vi "ExtractLoopsFromDrawI32WithSaveTST SAve2.vi"() -> ()   [LabVIEW 2018]
uses:
  <vilib>/vision/Image Controls.llb/IMAQ Image.ctl
  GlobalArrayLoops.vi
  <vilib>/vision/NI_Vision_Development_Module.lvlib
  <vilib>/ptbypt/NI_PtbyPt.lvlib
  <vilib>/Analysis/NI_AALBase.lvlib
panel:
  in  "Delay":dbl
  in  "AppendName":string
  in  "Constant":dbl=2.0 format="%.2f"
  in  "# Shifts":i32 min=0 max=8 step=1
  out "Image Out":T1
  in  "Initialize":bool
  in  "Image shift Y":i16
  in  "Image shift X":i16
  in  "Rot of image (deg)":sgl format="%.2f"
  in  "Normalize?":bool
  in  "Export All loops":bool
  in  "Shift Brightness?":bool
  in  "Enhance contrast?":bool
  in  "process loops?":bool=TRUE
  in  "Data Shift (bits)":i32=32768
  in  "Optional Rectangle":i32[](array[numeric])
  in  "Offset":dbl
  in  "SubtractBackground":bool
  in  "SaveBackground":bool
  in  "Save Button":bool
  out "CentersY":dbl[](array[numeric])
  out "CentersX":dbl[](array[numeric])
  in  "expAll":bool
  in  "exp":bool
  in  "contrast":dbl=1.0 format="%.2f"
  in  "Shift bright":dbl format="%.2f"
  out "ROI":T2
  out "Other Parameters":sgl[](array[numeric])
  out "Coordinates":i32[](array[numeric])
  in  "Loop stretch factor":dbl=15.0
  in  "Overlay loops!":bool
  out "Waveform Graph":dbl[][](graph)
  out "Coercive field  array":dbl[](array[numeric])
  out "Saturation array":dbl[](array[numeric])
  out "element":path
  out "BField":dbl[](array[numeric])
  in  "quadratic":dbl
  in  "Artificial x axis":bool
  in  "Faraday":dbl
  out "Remanence array":dbl[](array[numeric])=[-0.6665042042732239, -0.6516115069389343, -0.6760320067405701, -0.7227444648742676, 0.9848632216453552, 0.9883291125297546, 0.9750781655311584, 0.9934242963790894, 0.998292863368988, 0.9937769174575806, 0.9914392828941345, 0.9886137247085571, 0.9929239749908447, 0.9905381798744202, 0.988884687423706, 0.9859522581100464]
  out "ArrayLoops":dbl[][](array[numeric])=[[-8.399140210504821e+16, -6.383327329538546e+16, -7.300137106498384e+16, -7.299504888063269e+16, -7.545170145583659e+16, -6.992078814201549e+16, -8.44639172329355e+16, -1.3869430462570203e+17, -1.940946935865587e+17, -2.6899589959241552e+17, -3.841794265110722e+18, -3.5900544809762724e+18, -3.6362559596608225e+18, -3.50006165326631e+18, -3.327418536555498e+18, -3.784010531202494e+18, -3.449798578704159e+18, -3.328924867465459e+18, -3.311856048910509e+18, -3.4747904779405885e+18, -3.363990492336348e+18, -3.5235450226296233e+18, -3.5302608397729183e+18, -3.312218887780462e+18, -3.018598705633053e+18, -2.597754032832259e+18, -1.6360642472216494e+18, -1.0784516950489162e+17, -9.602954260961573e+16, -6.323074092330715e+16, -7.149779705137957e+16, -6.551521684505044e+16, -7.017147678836868e+16, -5.66990233766953e+16, -7.36723480449653e+16, 9.06092203023e-312, 2.141114181e-314, 2.4380364662986284e-231, 9.346337195181631e+20, 1.633936759043e-312, 8.184566024846808e-246, 3.441969216927865e-231, 1.8079404139024e-311, 5.8225571452e-313, 7.0610898928135075e-248, 5.749237705750308e-237, 2.80802498703826e-272, 4.45619116103e-313, 1.9118376e-316, 1.08168262e-315, 1.2469008049271105e+190, 5.335e-320, 3.18299368694e-313, 5.3527994774636694e+112, 1.4981290295104e-311, 1.6e-322, 2.1219957984e-314, 1.1251988247307957e-242, 3.1959050680695386e-231, 6.491120506e-315, 7.6391848542e-313, 2.3e-322, 1.455191297151144e-297, 2.1734535962868656e-66, 4.15911175029e-312, 5.995413155e-315, 3.18299368645e-313, 0.0, 1.1251988247307907e-242, 1.706694794319977e-138]]
  in  "n":i32=17
  out "XY Graph":cluster{"BField":dbl[], dbl[]}(graph)
  in  "Index of structure":i32
  in  "Array curves":dbl[][](array[numeric])=[[1.2468077718936927e+32, 1.1436107690770144e+32, 1.622459903179132e+32, 1.5181185795245691e+32, 2.0453528136560583e+32, 2.0512036276842735e+32, 2.9457901653443808e+32, 2.6269200225087976e+32, 1.193618727e-315, 2.1814116731123e-311, 1.032625499241048e-305, 7.46947828771e-312, 7.46942518498e-312, 8.1e-322, 8.289046e-317, 0.0]]
  out "Array":sgl[](array[numeric])=[20196.236, 20196.082, 20275.379, 20237.95, 19425.816, 19220.783, 19457.14, 19034.357, 18600.703, 18844.629, 18578.557, 18244.92, 17575.152, 17728.125, 17648.24, 17715.977]
  in  "Go through all images at one rot.":bool
  in  "stop":bool
  out "Image":T1(plugin-control)
  in  "index":i32(slide)=70 min=-1 max=160 step=1 scale=0.0..160.0
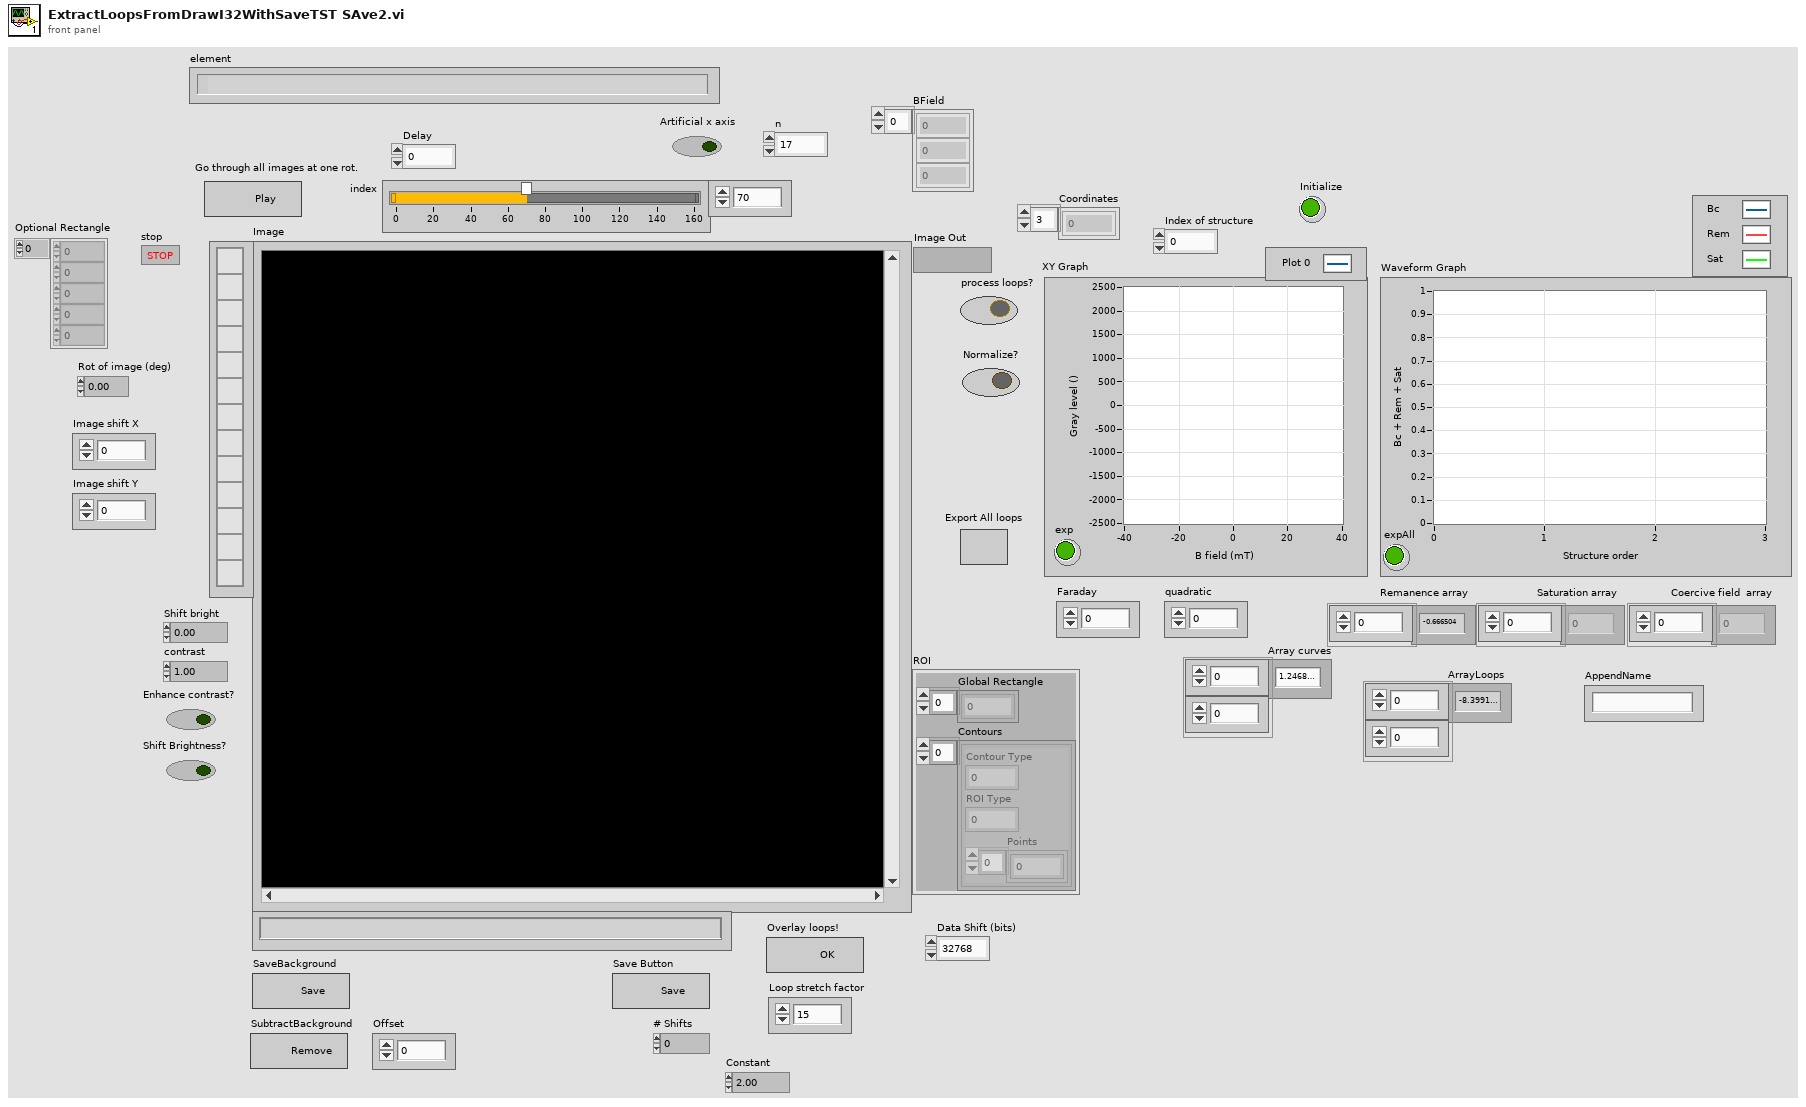
[diagram p1: front panel]
types:
  T1 = typedef "IMAQ Image.ctl" = refnum<image>
  T2 = cluster{"Global Rectangle":i32[], "Contours":cluster{"Contour Type":u32, "ROI Type":u32, "Points":i32[]}[]}
  T3 = typedef "Image Type" = u32
  T4 = cluster{"Desired Font (Application)":enum16{"User-specified Font", "Application Font", "System Font", "Dialog Font"}, "[User-specified Font]":cluster{"Font Name":string, "Size":i16, "Strikeout?":bool, "Italic?":bool, "Underline?":bool, "Outline?":bool, "Shadow?":bool, "Bold?":bool, "Rotation Angle":dbl}, "Horizontal Alignment":i16, "Vertical Alignment":i16}
  T5 = cluster{"Contour Type":u32, "ROI Type":u32, "Points":i32[]}[]
  T6 = cluster{"Global Rectangle":i32[], cluster{"Contour Type":u32, "ROI Type":u32, "Points":i32[]}[]}
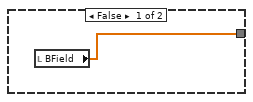
[diagram p6: hidden frame]
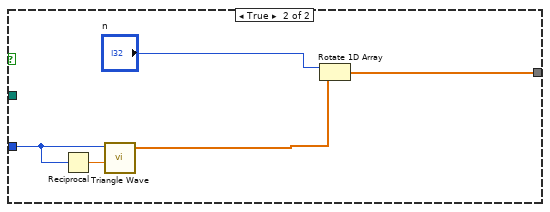
[diagram p7: hidden frame]
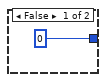
[diagram p9: hidden frame]
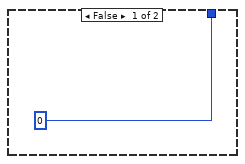
[diagram p13: hidden frame]
diagram:
  w5 = T3 1 items=["Grayscale (U8)", "Grayscale (I16)", "Grayscale (SGL)", "Complex (CSG)", "RGB (U32)", "HSL (U32)", "RGB (U64)", "Grayscale (U16)"] ("Image Type")
  w8 = T3 1 items=["Grayscale (U8)", "Grayscale (I16)", "Grayscale (SGL)", "Complex (CSG)", "RGB (U32)", "HSL (U32)", "RGB (U64)", "Grayscale (U16)"] ("Image Type")
  w12 = T3 1 items=["Grayscale (U8)", "Grayscale (I16)", "Grayscale (SGL)", "Complex (CSG)", "RGB (U32)", "HSL (U32)", "RGB (U64)", "Grayscale (U16)"] ("Image Type")
  w23 = T3 0 items=["Grayscale (U8)", "Grayscale (I16)", "Grayscale (SGL)", "Complex (CSG)", "RGB (U32)", "HSL (U32)", "RGB (U64)", "Grayscale (U16)"] ("Image Type")
  w26 = T3 7 items=["Grayscale (U8)", "Grayscale (I16)", "Grayscale (SGL)", "Complex (CSG)", "RGB (U32)", "HSL (U32)", "RGB (U64)", "Grayscale (U16)"] ("Image Type")
  n1 = call "File Dialog2"() -> ("selected path"=w18:path)  [unwired: 12 in, 3 out]
  n2 = disable-structure shown="Disabled" {
    disable-tunnel: [w33 _] -> _
    frame Disabled {
      n3 = call "File Dialog"() -> ("selected paths"=w33:path[])  [unwired: 12 in, 3 out]
    }
    frame Enabled {
    }
  }
  n4 = List Folder(path=w18, pattern="*.png") -> (path out=w17:path, filenames=w16:string[])  [unwired: 2 in, 2 out]
  n5 = for {
    tunnel: [w37] -> w15 mode=indexing if=w34
    tunnel: w17 -> [w38]
    tunnel: w16 -> [w36] mode=indexing
    n6 = Not Equal?(x=w36, y="mask.png") -> (x != y?=w34:bool)
    n7 = Build Path(base path=w38, name or relative path=w36) -> (appended path=w37:path)
  }
  n8 = Array Size(array=w15) -> (size(s)=w3:i32)
  n9 = List Folder(path=w18, pattern="*.txt") -> (path out=w13:path, filenames=w21:string[])  [unwired: 2 in, 2 out]
  n10 = Decrement(x=w3) -> (x-1=w1:i32)
  n11 = call "IMAQ Create"("Image Name"="sub", "Image Type"=w8) -> ("New Image"=w7:T1)  [unwired: 3 in, 1 out]
  n12 = property on="index" class="Slide (strict)"("Maximum"=w1) -> ()  [unwired: 2 in, 2 out]
  n13 = Index Array(array=w21) -> (element=w20:string)  [unwired: 1 in]
  n14 = property on="index" class="Slide (strict)"("Scale.Maximum"=w1) -> ()  [unwired: 2 in, 2 out]
  n15 = call "IMAQ Create"("Image Name"="Baxck", "Image Type"=w12) -> ("New Image"=w10:T1)  [unwired: 3 in, 1 out]
  n16 = Build Path(base path=w13, name or relative path=w20) -> (appended path=w19:path)
  n17 = call "IMAQ Create"("Image Name"="i32", "Image Type"=w5) -> ("New Image"=w2:T1)  [unwired: 3 in, 1 out]
  n18 = call "IMAQ Create"("Image Name"="a", "Image Type"=w26) -> ("New Image"=w32:T1, "error out"=w31:errorcluster)  [unwired: 3 in]
  n19 = call "IMAQ Create"("Image Name"="mask", "Image Type"=w23) -> ("New Image"=w25:T1)  [unwired: 3 in, 1 out]
  n20 = while {
    tunnel: w31 -> [w136]
    tunnel: [w107] -> w30
    tunnel: [w45] -> w28
    tunnel: w25 -> [w116]
    tunnel: [w115] -> w24
    tunnel: w15 -> [w108]
    tunnel: w19 -> [w100]
    tunnel: w3 -> [w46]
    tunnel: w13 -> [w56]
    tunnel: w10 -> [w73]
    tunnel: w7 -> [w68]
    tunnel: w2 -> [_]
    tunnel: w32 -> [w137]
    shift-right: [w43] -> _
    shift-left: w2 -> [w44]
    i -> [w98]
    stop <- "stop" stop-if-true
    w102 = 4 items=["None", "Selection Tool", "Point Tool", "Line Tool", "Rectangle Tool", "Oval Tool", "Polygon Tool", "ClosedFreehandTool", "Annulus Tool", "Rotated Rectangle Tool", "Zoom Tool", "Pan Tool", "Polyline Tool", "Freehand Tool"] ("Tool")
    w124 = i32[] [2] items=["No Event"=0, "Click Event"=1, "Draw Event"=2, "Size Event"=4, "Scroll Event"=5, "Double Click Event"=8] ("Which Events")
    n21 = Equal To 0?(x=w98) -> (x = 0?=w97:bool)
    n22 = case shown="False" "Artificial x axis" {
      tunnel: [w164 w183] -> w55
      tunnel: w100 -> [w165 _]
      tunnel: w97 -> [w163 _]
      tunnel: w46 -> [_ w182]
      frame False {
        n23 = case shown="True" w163 {
          tunnel: w165 -> [_ w171]
          tunnel: [w166 w169] -> w164
          frame False {
            n24 = local read "BField"() -> (w166:dbl[])
          }
          frame True {
            n25 = Read from Text File(file (use dialog)=w171) -> (text=w173:string)  [unwired: 3 in, 3 out]
            n26 = Search and Replace String(replace all?=TRUE ("replace all? (F)"), input string=w173, search string=".", replace string="," ("replace string (\"\")")) -> (result string=w167:string)  [unwired: 4 in, 3 out]
            n27 = Spreadsheet String To Array(format string="%.6f", spreadsheet string=w167) -> (array=w177:dbl[][])  [unwired: 2 in]
            n28 = Array Size(array=w177) -> (size(s)=w178:i32[])
            n29 = Index Array(array=w178) -> (element=w180:i32)  [unwired: 1 in]
            n30 = Array Subset(array=w177, index (row)=1 ("index"), length (row)=w180, length (col)=2 ("length")) -> (w170:dbl[][])  [unwired: 1 in]
            n31 = Index Array(array=w170, index (col)=0 ("disabled index (col)")) -> (element=w169:dbl[])  [unwired: 1 in]
            "BField" <- w169
          }
        }
      }
      frame True {
        n32 = Reciprocal(x=w182) -> (1/x=w186:dbl)
        n33 = call <vilib>:"Triangle Wave.vi"("samples"=w182, "frequency"=w186) -> ("triangle wave"=w185:dbl[])  [unwired: 3 in, 2 out]
        n34 = Rotate 1D Array(1:w185, 2:"n") -> (0:w183:dbl[])
      }
    }
    n35 = local read "Array curves"() -> (w63:dbl[][])
    n36 = invoke on="Image" class="ImageControl" method="Get Last Event"("Which Events"=w124) -> ("Tool"=w103:i32, "Coordinates"=w122:i32[], "Other Parameters"=w82:sgl[])  [unwired: 7 in, 5 out]
    n37 = Array Size(array=w63) -> (size(s)=w113:i32[])
    n38 = Empty Array?(array=w122) -> (empty?=w121:bool)
    n39 = feedback #1() -> (w123:i32[])  [unwired: 1 in]
    n40 = feedback-in #1(w122) -> ()
    n41 = Index Array(array=w113, index=1) -> (element=w111:i32)
    n42 = Not Equal?(x=w122, y=w123) -> (x != y?=w120:bool)
    n43 = Not(x=w121) -> (.not. x?=w119:bool)
    n44 = feedback #2() -> (w134:bool)  [unwired: 1 in]
    n45 = feedback-in #2("Go through all images at one rot.") -> ()
    n46 = Not Equal?(x="Go through all images at one rot.", y=w134) -> (x != y?=w105:bool)
    n47 = for {
      N: w111 -> [_]
      tunnel: w55 -> [w203]
      tunnel: w63 -> [w242]
      shift-right: [w238] -> _
      shift-left: sgl 0.0 -> [w241]
      tunnel: [w240] -> _ mode=indexing
      tunnel: [w191] -> w66 mode=indexing
      tunnel: [w231] -> w93 mode=indexing
      tunnel: "Faraday" -> [w227]
      tunnel: "quadratic" -> [w224]
      tunnel: [w212] -> w89 mode=indexing
      tunnel: [w204] -> w96 mode=indexing
      tunnel: w46 -> [w201]
      tunnel: "Normalize?" -> [w190]
      i -> [w243]
      n48 = Square(x=w203) -> (x^2=w222:dbl[])
      n49 = Multiply(x=w222, y=w224) -> (x*y=w225:dbl[])
      n50 = Absolute Value(x=w203) -> (abs(x)=w202:dbl[])
      n51 = Divide(x=w201, y=4) -> (x/y=w213:dbl)
      n52 = Multiply(x=w203, y=w227) -> (x*y=w221:dbl[])
      n53 = Index Array(array=w242, index (col)=w243) -> (element=w193:dbl[])  [unwired: 1 in]
      n54 = Array Size(array=w193) -> (size(s)=w194:i32)
      n55 = Decrement(x=w194) -> (x-1=w195:i32)
      n56 = Index Array(array=w193, index #1=0, index #2=w195) -> (element #1=w198:dbl, element #2=w199:dbl)
      n57 = Subtract(x=w199, y=w198) -> (x-y=w197:dbl)
      n58 = Divide(x=w197, y=w194) -> (x/y=w196:dbl)
      n59 = for {
        tunnel: w193 -> [w246] mode=indexing
        tunnel: w196 -> [w247]
        tunnel: [w244] -> w192 mode=indexing
        i -> [w248]
        n60 = Multiply(x=w247, y=w248) -> (x*y=w245:dbl)
        n61 = Subtract(x=w246, y=w245) -> (x-y=w244:dbl)
      }
      n62 = Array Max & Min(array=w192) -> (min value=w239:dbl)  [unwired: 3 out]
      n63 = Array Max & Min(array=w192) -> (max value=w229:dbl, min value=w235:dbl)  [unwired: 2 out]
      n64 = Subtract(x=w192, y=w239) -> (x-y=w237:dbl[])
      n65 = Add(x=w229, y=w235) -> (x+y=w234:dbl)
      n66 = Add(x=w237, y=w241) -> (x+y=w236:dbl[])
      n67 = Divide(x=w234, y=sgl 2.0) -> (x/y=w232:dbl)
      n68 = Subtract(x=w192, y=w232) -> (x-y=w226:dbl[])
      n69 = Array Max & Min(array=w236) -> (max value=w238:dbl)  [unwired: 3 out]
      n70 = Add(x=w225, y=w226) -> (x+y=w223:dbl[])
      n71 = Add(x=w221, y=w223) -> (x+y=w215:dbl[])
      n72 = Array Max & Min(array=w215) -> (max value=w220:dbl, min value=w219:dbl)  [unwired: 2 out]
      n73 = Add(x=w220, y=w219) -> (x+y=w217:dbl)
      n74 = Divide(x=w217, y=sgl 2.0) -> (x/y=w216:dbl)
      n75 = Subtract(x=w215, y=w216) -> (x-y=w189:dbl[])
      n76 = Array Max & Min(array=w189) -> (max value=w212:dbl)  [unwired: 3 out]
      n77 = Index Array(array=w189, index=w213) -> (element=w230:dbl)
      n78 = Array Max & Min(array=w189) -> (max value=w228:dbl)  [unwired: 3 out]
      n79 = for {
        tunnel: w189 -> [w253] mode=indexing
        tunnel: [w251] -> w211 mode=indexing if=w250
        i -> [w251]
        n80 = Equal To 0?(x=w251) -> (x = 0?=w252:bool)
        n81 = call <vilib>:"Zero Crossing PtByPt.vi"("initialize"=w252, "direction"=enum16{"either", "minus-plus", "plus-minus"}."either", "input data point"=w253) -> ("crossing"=w250:bool)
      }
      n82 = Divide(x=w230, y=w228) -> (x/y=w231:dbl)
      n83 = Array Max & Min(array=w189) -> (max value=w188:dbl)  [unwired: 3 out]
      n84 = Index Array(array=w211) -> (element #1=w210:i32, element #2=w209:i32)  [unwired: 2 in]
      n85 = Divide(x=w189, y=w188) -> (x/y=w187:dbl[])
      n86 = Index Array(array=w202, index #1=w210, index #2=w209) -> (element #1=w207:dbl, element #2=w208:dbl)
      n87 = Add(x=w207, y=w208) -> (x+y=w206:dbl)
      n88 = Select(t=w187, s=w190, f=w189) -> (s? t:f=w191:dbl[])
      n89 = Divide(x=w206, y=2.0) -> (x/y=w204:dbl)
      n90 = Bundle("BField"=w203, w236) -> (w240:cluster{"BField":dbl[], dbl[]})  [unwired: 1 in]
    }
    "ArrayLoops" <- w66
    "Remanence array" <- w93
    "Saturation array" <- w89
    "Coercive field  array" <- w96
    n91 = Select(t=u32 10, s="Go through all images at one rot.", f=u32 400 ("milliseconds to wait")) -> (s? t:f=w127:u32)
    n92 = Equal?(x=w103, y=w102) -> (x = y?=w104:bool)
    n93 = Compound Arithmetic op=AND(w104, w120, w119) -> (w118:bool)
    n94 = case shown="True" w118 {
      tunnel: w122 -> [_ w263]
      tunnel: w82 -> [_ w260]
      tunnel: w46 -> [_ w255]
      frame False {
      }
      frame True {
        n95 = property on="Image" class="ImageControl"() -> ("ROI"=w258:T2)  [unwired: 2 in, 2 out]
        "ROI" <- w258
        n96 = Index Array(array=w263, index #1=0 ("index"), index #2=1 ("index")) -> ()  [unwired: 2 out]
        n97 = Unbundle(w258) -> ("Contours"=w257:T5)  [unwired: 1 out]
        n98 = Array Size(array=w257) -> (size(s)=w254:i32)
        n99 = Initialize Array(0.0, w255, w254) -> (w256:dbl[][])
        n100 = local write "Array curves"(w256) -> ()
        "Coordinates" <- w263
        "Other Parameters" <- w260
      }
    }
    n101 = And(x="Go through all images at one rot.", y=w105) -> (x .and. y?=w131:bool)
    n102 = Wait (ms)(milliseconds to wait=w127) -> ()  [unwired: 1 out]
    n103 = case shown="True" w131 {
      tunnel: [0 ("index") w266] -> w133
      frame False {
      }
      frame True {
        w266 = 0 ("index")
        n104 = local write "index"(w266) -> ()
        n105 = property on="index" class="Slide (strict)"("Val(Sgnl)"=w266) -> ()  [unwired: 2 in, 2 out]
      }
    }
    n106 = flat-sequence {
      tunnel: ["index"] -> w117
      tunnel: w133 -> [_]
      frame #0 {
      }
    }
    n107 = case shown="True" "Initialize" {
      tunnel: w46 -> [_ w139]
      frame False {
      }
      frame True {
        n108 = local read "Array curves"() -> (w144:dbl[][])
        n109 = Array Size(array=w144) -> (size(s)=w143:i32[])
        n110 = Index Array(array=w143, index #2=1 ("index")) -> (element #2=w142:i32)  [unwired: 1 in, 1 out]
        n111 = Initialize Array(0.0, w139, w142) -> (w140:dbl[][])
        n112 = local write "Array curves"(w140) -> ()
      }
    }
    n113 = Transpose 2D Array(2D array=w63) -> (transposed array=w64:dbl[][])
    n114 = Bundle("index"=w117) -> (w84:cluster{"index":i32})  [unwired: 1 in]
    n115 = Increment(x=w117) -> (x+1=w126:i32)
    n116 = Select(t=w66, s="process loops?", f=w64) -> (s? t:f=w53:dbl[][])
    n117 = Increment(x=w126) -> (x+1=w125:i32)
    n118 = Index Array(array=w53, index (row)="Index of structure") -> (element=w54:dbl[])  [unwired: 1 in]
    n119 = feedback-in #3(w84) -> ()
    n120 = feedback #3() -> (w85:cluster{"index":i32})  [unwired: 1 in]
    n121 = local read "Index of structure"() -> (w77:i32)
    n122 = Not Equal?(x=w84, y=w85) -> (x != y?=w132:bool)
    n123 = Greater Or Equal?(x=w125, y=w46) -> (x >= y?=w130:bool)
    n124 = global write "GlobalArrayLoops.vi" "Array loops"(w66) -> ()
    n125 = global write "GlobalArrayLoops.vi" "B field (mT)"(w55) -> ()
    n126 = Bundle("BField"=w55, w54) -> (→"XY Graph":cluster{"BField":dbl[], dbl[]})  [unwired: 1 in]
    n127 = Or(x=w131, y=w132) -> (x .or. y?=w59:bool)
    n128 = case shown="True" "exp" {
      tunnel: w56 -> [_ w146]
      tunnel: w77 -> [_ w159]
      frame False {
      }
      frame True {
        n129 = Build Path(base path=w146, name or relative path="exp") -> (appended path=w148:path)
        n130 = call <vilib>:"Check if File or Folder Exists.vi"("path"=w148) -> ("file or folder exists?"=w149:bool, "dup path"=w150:path)  [unwired: 8 in, 1 out]
        n131 = case shown="False" w149 {
          tunnel: w150 -> [w161 w162]
          tunnel: [w160 w162] -> w145
          frame False {
            n132 = Create Folder(path (use dialog)=w161) -> (created path=w160:path)  [unwired: 2 in, 2 out]
          }
          frame True {
          }
        }
        n133 = Number To Decimal String(number=w159) -> (decimal integer string=w158:string)  [unwired: 1 in]
        n134 = Concatenate Strings("LoopStrucNo_" ("string"), w158, ".bmp" ("string")) -> (w155:string)
        n135 = Build Path(base path=w145, name or relative path=w155) -> (appended path=w154:path)
        n136 = invoke on="XY Graph" class="XYGraph (strict)" method="Export Image"("FileType"=enum32{"BMP", "EPS", "EMF", "PICT"}."BMP" ("File Type"), "Target"=enum32{"File", "Clipboard"}."File", "Path"=w154, "HideGrid"=TRUE ("Hide Grid")) -> ()  [unwired: 4 in, 8 out]
      }
    }
    n137 = case shown="True" w130 {
      frame False {
      }
      frame True {
        n138 = local write "Go through all images at one rot."(FALSE ("Go through all")) -> ()
      }
    }
    n139 = Absolute Value(x=w96) -> (abs(x)=w41:dbl[])
    n140 = Absolute Value(x=w89) -> (abs(x)=w39:dbl[])
    n141 = Absolute Value(x=w93) -> (abs(x)=w40:dbl[])
    n142 = Array Max & Min(array=w41) -> (max value=w95:dbl)  [unwired: 3 out]
    n143 = Array Max & Min(array=w39) -> (max value=w90:dbl)  [unwired: 3 out]
    n144 = Array Max & Min(array=w40) -> (max value=w94:dbl)  [unwired: 3 out]
    n145 = Divide(x=w41, y=w95) -> (x/y=w92:dbl[])
    n146 = Divide(x=w39, y=w90) -> (x/y=w88:dbl[])
    n147 = Divide(x=w40, y=w94) -> (x/y=w91:dbl[])
    n148 = Array Size(array=w53) -> (size(s)=w52:i32[])
    n149 = Index Array(array=w52) -> (element=w51:i32)  [unwired: 1 in]
    n150 = Build Array(w92, w91, w88) -> (w42:dbl[][])
    "Waveform Graph" <- w42
    n151 = case shown="True" "expAll" {
      tunnel: w56 -> [_ w486]
      tunnel: w42 -> [_ _]
      tunnel: w41 -> [_ w466]
      tunnel: w40 -> [_ w465]
      tunnel: w39 -> [_ w464]
      frame False {
      }
      frame True {
        w474 = "\t"
        n152 = Build Path(base path=w486, name or relative path="exp") -> (appended path=w484:path)
        n153 = call <vilib>:"Check if File or Folder Exists.vi"("path"=w484) -> ("file or folder exists?"=w483:bool, "dup path"=w482:path)  [unwired: 8 in, 1 out]
        n154 = case shown="False" w483 {
          tunnel: w482 -> [w495 w496]
          tunnel: [w494 w496] -> w468
          frame False {
            n155 = Create Folder(path (use dialog)=w495) -> (created path=w494:path)  [unwired: 2 in, 2 out]
          }
          frame True {
          }
        }
        n156 = Build Array(w466, w465, w464) -> (w463:dbl[][])
        n157 = local read "AppendName"() -> (w479:string)
        n158 = Transpose 2D Array(2D array=w463) -> (transposed array=w481:dbl[][])
        n159 = Array To Spreadsheet String(array=w481, 3:"%.6f" ("format string")) -> (spreadsheet string=w477:string)  [unwired: 1 in]
        n160 = Concatenate Strings("ExportAll" ("string"), ".bmp" ("string")) -> (w492:string)
        n161 = Concatenate Strings("ExportGraphData" ("name or relative path"), w479, ".txt" ("string")) -> (w470:string)
        n162 = Concatenate Strings("Bc (mT)" ("name or relative path"), w474, "Rem ()" ("name or relative path"), w474, "Sat (...)" ("name or relative path"), "\r\n", w477) -> (w469:string)
        n163 = Build Path(base path=w468, name or relative path=w492) -> (appended path=w490:path)
        n164 = Build Path(base path=w468, name or relative path=w470) -> (appended path=w467:path)
        n165 = invoke on="Waveform Graph" class="WFGraph (strict)" method="Export Image"("FileType"=enum32{"BMP", "EPS", "EMF", "PICT"}."BMP" ("File Type"), "Target"=enum32{"File", "Clipboard"}."File", "Path"=w490, "HideGrid"=TRUE ("Hide Grid")) -> ()  [unwired: 4 in, 8 out]
        n166 = Write to Text File(file (use dialog)=w467, text=w469) -> ()  [unwired: 2 in, 3 out]
      }
    }
    n167 = case shown="True" w59 {
      tunnel: w137 -> [_ w277]
      tunnel: w136 -> [w270 w306]
      tunnel: w117 -> [_ w292]
      tunnel: [w270 w285] -> w107
      tunnel: [w268 w302] -> w87
      tunnel: w116 -> [w269 w300]
      tunnel: [w269 w299] -> w115
      tunnel: w108 -> [_ w295]
      tunnel: w44 -> [w268 w282]
      tunnel: "Image shift X" -> [_ w272]
      tunnel: "Image shift Y" -> [_ w271]
      frame False {
      }
      frame True {
        n168 = local read "ROI"() -> (w289:T2)
        n169 = Index Array(array=w295, index=w292) -> (element=w294:path)
        "element" <- w294
        n170 = call "IMAQ ReadFile"("File Path"=w294, "error in (no error)"=w306, "Image"=w277) -> ("Image Out"=w276:T1)  [unwired: 4 in, 4 out]
        n171 = call "IMAQ Rotate"("Maintain Size"=FALSE, "Angle (degrees)"="Rot of image (deg)", "Image Src"=w276) -> ("Image Dst Out"=w274:T1)  [unwired: 7 in, 1 out]
        n172 = Unbundle(w289) -> ("Global Rectangle"=w290:i32[], "Contours"=w291:T5)
        n173 = call "IMAQ Shift"("YOffset"=w271, "XOffset"=w272, "Image Src"=w274) -> ("Image Dst Out"=w273:T1)  [unwired: 7 in, 1 out]
        n174 = case shown="True" TRUE {
          tunnel: w282 -> [_ w312]
          tunnel: [w307 w311] -> w281
          tunnel: w273 -> [w307 w308]
          frame False {
          }
          frame True {
            n175 = call "IMAQ ImageToArray"("Optional Rectangle"="Optional Rectangle", "Image"=w308) -> ("Image Pixels (U16)"=w316:u16[][])  [unwired: 2 in, 4 out]
            n176 = To Long Integer(number=w316) -> (32bit integer=w315:i32[][])
            n177 = Subtract(x=w315, y="Data Shift (bits)") -> (x-y=w313:i32[][])
            n178 = To Word Integer(number=w313) -> (16bit integer=w310:i16[][])
            n179 = call "IMAQ ArrayToImage"("Image Pixels (I16)"=w310, "Image"=w312) -> ("Image Out"=w311:T1)  [unwired: 8 in, 1 out]
          }
        }
        n180 = Wait (ms)(milliseconds to wait="Delay") -> ()  [unwired: 1 out]
        n181 = call "IMAQ Clear Overlay"("Groups"=string[] ["Circ"], "Image"=w281) -> ("error out"=w304:errorcluster, "Image Out"=w303:T1)  [unwired: 8 in]
        n182 = Array Size(array=w290) -> (size(s)=w287:i32)
        n183 = Initialize Array(u32 16712704 ("Color (red)"), w287) -> (w286:u32[])
        n184 = call <vilib>:"Clear Errors.vi"("error in (no error)"=w304) -> ("error out"=w301:errorcluster)  [unwired: 5 in, 1 out]
        n185 = for {
          shift-right: [w328] -> w302
          shift-left: w303 -> [w340]
          shift-right: [w352] -> w285
          shift-left: w301 -> [w351]
          tunnel: [w350] -> w293 mode=indexing
          shift-right: [w349] -> w299
          shift-left: w300 -> [w348]
          tunnel: w290 -> [w344]
          tunnel: w291 -> [w339] mode=indexing
          tunnel: w286 -> [w347]
          tunnel: [w321] -> w284 mode=indexing
          tunnel: [w320] -> w283 mode=indexing
          i -> [w326]
          w330 = 2.0
          w327 = "Circ" ("Group")
          n186 = Build Array(w339) -> (w345:T5)
          n187 = Unbundle(w339) -> ("Points"=w337:i32[])  [unwired: 2 out]
          n188 = Bundle("Global Rectangle"=w344, w345) -> (w343:T6)  [unwired: 1 in]
          n189 = Index Array(array=w337, index #1=2 ("index"), index #2=0 ("index"), index #3=3 ("index"), index #4=1 ("index")) -> (element #1=w332:i32, element #2=w319:i32, element #3=w318:i32, element #4=w317:i32)
          n190 = Add(x=w332, y=w319) -> (x+y=w322:i32)
          n191 = Add(x=w318, y=w317) -> (x+y=w331:i32)
          n192 = Divide(x=w331, y=w330) -> (x/y=w320:dbl)
          n193 = Divide(x=w322, y=w330) -> (x/y=w321:dbl)
          n194 = Number To Decimal String(number=w326) -> (decimal integer string=w325:string)  [unwired: 1 in]
          n195 = Bundle(w319, w317) -> (w329:cluster{i32, i32})  [unwired: 1 in]
          n196 = call "IMAQ Overlay ROI"("Colors (Green)"=w347, "Group"=w327, "error in (no error)"=w351, "ROI Descriptor"=w343, "Image"=w340) -> ("error out"=w352:errorcluster, "Image Out"=w338:T1)  [unwired: 5 in]
          n197 = call "IMAQ Overlay Text"("Group"=w327, "Text Color (black)"=u32 0, "Font, Size & Style"=T4 {"Desired Font (Application)"=enum."User-specified Font", "[User-specified Font]"={"Font Name"="", "Size"=16, "Strikeout?"=FALSE, "Italic?"=FALSE, "Underline?"=FALSE, "Outline?"=FALSE, "Shadow?"=FALSE, "Bold?"=FALSE, "Rotation Angle"=0.0}, "Horizontal Alignment"=0, "Vertical Alignment"=1}, "String"=w325, "Origin"=w329, "Image"=w338) -> ("Image Out"=w328:T1)  [unwired: 4 in, 1 out]
          n198 = call "IMAQ ROIToMask 2"("Image Model"=w328, "Filling Value (255)"=255, "ROI Descriptor"=w343, "Image"=w348) -> ("error out"=w342:errorcluster, "Image Out"=w349:T1)  [unwired: 5 in, 1 out]
          n199 = call "IMAQ Histograph"("error in (no error)"=w342, "Image Mask"=w349, "Image"=w328) -> ("error out"=w341:errorcluster, "Mean Value"=w350:sgl)  [unwired: 5 in, 2 out]
          n200 = call <vilib>:"Clear Errors.vi"("error in (no error)"=w341) -> ()  [unwired: 5 in, 2 out]
        }
        "Array" <- w293
        "CentersX" <- w284
        "CentersY" <- w283
        n201 = local read "index"() -> (w297:i32)
        n202 = Replace Array Subset(array="Array curves", new element=w293, index (row)=w297) -> (w296:dbl[][])  [unwired: 1 in]
        n203 = invoke on="Image" class="ImageControl" method="Clear ROI"(error in=w285) -> ()  [unwired: 2 in, 3 out]
        n204 = local write "Array curves"(w296) -> ()
      }
    }
    n205 = case shown="True" "Export All loops" {
      tunnel: w54 -> [_ w364]
      tunnel: w55 -> [_ w365]
      tunnel: w51 -> [_ w366]
      tunnel: w56 -> [_ w355]
      tunnel: [0 w362] -> _
      frame False {
      }
      frame True {
        n206 = flat-sequence {
          tunnel: w366 -> [w372]
          tunnel: w365 -> [w383]
          tunnel: w364 -> [w382]
          tunnel: [w381] -> w363
          tunnel: [w376] -> w361
          tunnel: [w373] -> w360
          tunnel: w363 -> [w396]
          tunnel: w361 -> [w394]
          tunnel: w360 -> [w389]
          tunnel: w354 -> [w386]
          tunnel: [w403] -> w362
          frame #0 {
            n207 = local read "Index of structure"() -> (w378:i32)
            n208 = Number To Decimal String(number=w378) -> (decimal integer string=w379:string)  [unwired: 1 in]
            n209 = Decrement(x=w372) -> (x-1=w371:i32)
            n210 = Concatenate Strings("ExportHysterplot" ("string"), "_Struc_" ("string"), w379) -> (w375:string)
            n211 = Less?(x=w378, y=w371) -> (x < y?=w385:bool)
            n212 = local write "Export All loops"(w385) -> ()
            n213 = Concatenate Strings(w375, ".txt" ("string")) -> (w376:string)
            n214 = Build Array(w383, w382) -> (w384:dbl[][])
            n215 = Concatenate Strings(w375, ".bmp" ("string")) -> (w373:string)
            n216 = Transpose 2D Array(2D array=w384) -> (transposed array=w381:dbl[][])
          }
          frame #1 {
            w393 = TRUE ("Always Overwrite")
            n217 = Build Path(base path=w386, name or relative path=w394) -> (appended path=w390:path)
            n218 = Array To Spreadsheet String(array=w396, 3:"%.6f" ("format string")) -> (spreadsheet string=w397:string)  [unwired: 1 in]
            n219 = Build Path(base path=w386, name or relative path=w389) -> (appended path=w388:path)
            n220 = Concatenate Strings("B field (mT)" ("name or relative path"), "\t", "Grey level ()" ("name or relative path"), "\r\n", w397) -> (w395:string)
            n221 = control-ref of="XY Graph"() -> (w387:refnum<vi>)
            n222 = invoke on="Invoke Node" class="XYGraph (strict)" method="Export Image"(reference=w387, "FileType"=enum32{"BMP", "EPS", "EMF", "PICT"}."BMP" ("File Type"), "Target"=enum32{"File", "Clipboard"}."File", "Path"=w388, "HideGrid"=w393, "Overwrite"=w393) -> ()  [unwired: 2 in, 8 out]
            n223 = Write to Text File(file (use dialog)=w390, text=w395) -> ()  [unwired: 2 in, 3 out]
          }
          frame #2 {
            n224 = local read "Index of structure"() -> (w404:i32)
            n225 = Increment(x=w404) -> (x+1=w403:i32)
            n226 = local write "Index of structure"(w403) -> ()
          }
        }
        n227 = Build Path(base path=w355, name or relative path="exp") -> (appended path=w357:path)
        n228 = call <vilib>:"Check if File or Folder Exists.vi"("path"=w357) -> ("file or folder exists?"=w358:bool, "dup path"=w359:path)  [unwired: 8 in, 1 out]
        n229 = case shown="False" w358 {
          tunnel: w359 -> [w368 w369]
          tunnel: [w367 w369] -> w354
          frame False {
            n230 = Create Folder(path (use dialog)=w368) -> (created path=w367:path)  [unwired: 2 in, 2 out]
          }
          frame True {
          }
        }
      }
    }
    n231 = case shown="True" "Overlay loops!" {
      tunnel: w87 -> [w505 w509]
      tunnel: [w505 w510] -> w45
      tunnel: w55 -> [_ w513]
      frame False {
      }
      frame True {
        n232 = local read "ArrayLoops"() -> (w508:dbl[][])
        n233 = local read "CentersX"() -> (w507:dbl[])
        n234 = local read "CentersY"() -> (w506:dbl[])
        n235 = Array Max & Min(array=w513) -> (max value=w512:dbl)  [unwired: 3 out]
        n236 = Divide(x=w513, y=w512) -> (x/y=w511:dbl[])
        n237 = call "IMAQ Clear Overlay"("Groups"=string[] ["Loops"], "Image"=w509) -> ("error out"=w514:errorcluster, "Image Out"=w516:T1)  [unwired: 8 in]
        n238 = call <vilib>:"Clear Errors.vi"("error in (no error)"=w514) -> ("error out"=w515:errorcluster)  [unwired: 5 in, 1 out]
        n239 = for {
          tunnel: w516 -> [w525]
          tunnel: w515 -> [_]
          tunnel: w508 -> [w518]
          tunnel: w511 -> [w534]
          tunnel: [w523] -> w510
          tunnel: w508 -> [_] mode=indexing
          tunnel: w507 -> [w520] mode=indexing
          tunnel: w506 -> [w519] mode=indexing
          i -> [w527]
          n240 = Index Array(array=w518, index (row)=w527) -> (element=w536:dbl[])  [unwired: 1 in]
          n241 = Array Max & Min(array=w518) -> (max value=w535:dbl)  [unwired: 3 out]
          n242 = Divide(x=w536, y=w535) -> (x/y=w532:dbl[])
          n243 = Multiply(x=w532, y="Loop stretch factor") -> (x*y=w531:dbl[])
          n244 = Multiply(x=w534, y="Loop stretch factor") -> (x*y=w533:dbl[])
          n245 = Add(x=w520, y=w533) -> (x+y=w530:dbl[])
          n246 = Add(x=w519, y=w531) -> (x+y=w529:dbl[])
          n247 = for {
            tunnel: w530 -> [w539] mode=indexing
            tunnel: w529 -> [w538] mode=indexing
            tunnel: [w537] -> w526 mode=indexing
            n248 = Bundle(w539, w538) -> (w537:cluster{dbl, dbl})  [unwired: 1 in]
          }
          n249 = call "IMAQ Overlay Multiple Lines 2"("Image"=w525, "Group"="Loops", "Line End Points"=w526, "Color"=u32 1245006, "Width"=u32 1) -> ("Image Out"=w523:T1)  [unwired: 9 in, 1 out]
        }
      }
    }
    n250 = And(x="Shift Brightness?", y=w59) -> (x .and. y?=w60:bool)
    n251 = case shown="True" w60 {
      tunnel: w45 -> [w501 w504]
      tunnel: "Shift bright" -> [_ w503]
      tunnel: [w501 w502] -> w81
      frame False {
      }
      frame True {
        n252 = call "IMAQ Subtract"("Image Src A"=w504, "Constant"=w503, "Image Dst"=w504) -> ("Image Dst Out"=w502:T1)  [unwired: 4 in, 1 out]
      }
    }
    n253 = And(x="Enhance contrast?", y=w59) -> (x .and. y?=w61:bool)
    n254 = case shown="True" w61 {
      tunnel: w81 -> [w497 w500]
      tunnel: [w497 w499] -> w72
      tunnel: "contrast" -> [_ w498]
      frame False {
      }
      frame True {
        n255 = call "IMAQ Multiply"("Image Src A"=w500, "Constant"=w498, "Image Dst"=w500) -> ("Image Dst Out"=w499:T1)  [unwired: 4 in, 1 out]
      }
    }
    n256 = case shown="True" "Go through all images at one rot." {
      tunnel: w107 -> [_ _]
      frame False {
      }
      frame True {
        n257 = local read "index"() -> (w541:i32)
        n258 = Increment(x=w541) -> (x+1=w540:i32)
        n259 = local write "index"(w540) -> ()
      }
    }
    n260 = case shown="True" "SaveBackground" {
      tunnel: w72 -> [_ w414]
      tunnel: w73 -> [w411 w413]
      tunnel: [w411 w412] -> w70
      tunnel: "Offset" -> [_ _]
      frame False {
      }
      frame True {
        n261 = call "IMAQ Copy"("Image Dst"=w413, "Image Src"=w414) -> ("Image Dst Out"=w412:T1)  [unwired: 4 in, 1 out]
      }
    }
    n262 = case shown="True" "SubtractBackground" {
      tunnel: w72 -> [w405 w408]
      tunnel: [w405 w406] -> w71
      tunnel: w70 -> [_ w410]
      tunnel: w68 -> [_ w409]
      tunnel: "Offset" -> [_ w407]
      frame False {
      }
      frame True {
        n263 = call "IMAQ Subtract"("Image Src A"=w408, "Constant"=w407, "Image Dst"=w409, "Image Src B"=w410) -> ("Image Dst Out"=w406:T1)  [unwired: 3 in, 1 out]
      }
    }
    "Image" <- w71
    n264 = case shown="True" "Save Button" {
      tunnel: w45 -> [w415 w430]
      tunnel: w56 -> [_ w451]
      tunnel: [w415 w430] -> w43
      frame False {
      }
      frame True {
        w429 = string[] ["Circ", "Loops"]
        w432 = T3 0 items=["Grayscale (U8)", "Grayscale (I16)", "Grayscale (SGL)", "Complex (CSG)", "RGB (U32)", "HSL (U32)", "RGB (U64)", "Grayscale (U16)"] ("Image Type")
        w434 = T3 0 items=["Grayscale (U8)", "Grayscale (I16)", "Grayscale (SGL)", "Complex (CSG)", "RGB (U32)", "HSL (U32)", "RGB (U64)", "Grayscale (U16)"] ("Image Type")
        w436 = u16 0 items=["RGB", "HSL", "HSV", "HSI"] ("Color Mode")
        (unwired) u16 0 items=["RGB", "HSL", "HSV", "HSI"] ("Color Mode")
        w443 = T3 7 items=["Grayscale (U8)", "Grayscale (I16)", "Grayscale (SGL)", "Complex (CSG)", "RGB (U32)", "HSL (U32)", "RGB (U64)", "Grayscale (U16)"] ("Image Type")
        w449 = T3 4 items=["Grayscale (U8)", "Grayscale (I16)", "Grayscale (SGL)", "Complex (CSG)", "RGB (U32)", "HSL (U32)", "RGB (U64)", "Grayscale (U16)"] ("Image Type")
        n265 = call "IMAQ Create"("Image Name"="Saveu8", "Image Type"=w434) -> ("New Image"=w426:T1)  [unwired: 3 in, 1 out]
        n266 = Build Path(base path=w451, name or relative path="exp") -> (appended path=w453:path)
        n267 = call <vilib>:"Check if File or Folder Exists.vi"("path"=w453) -> ("file or folder exists?"=w454:bool, "dup path"=w455:path)  [unwired: 8 in, 1 out]
        n268 = call "IMAQ GetImageSize"("Image"=w430) -> ("Y Resolution"=w439:i32, "X Resolution"=w438:i32)  [unwired: 3 in, 1 out]
        n269 = call "IMAQ Create"("Image Name"="Save", "Image Type"=w449) -> ("New Image"=w424:T1)  [unwired: 3 in, 1 out]
        n270 = call "IMAQ Create"("Image Name"="Saveu16", "Image Type"=w443) -> ("New Image"=w425:T1)  [unwired: 3 in, 1 out]
        n271 = Initialize Array(u32 0 ("element"), w439, w438) -> (w440:u32[][])
        n272 = call "IMAQ SetImageSize"("Y Resolution"=w439, "X Resolution"=w438, "Image"=w424) -> ("Image Out"=w442:T1)  [unwired: 2 in, 1 out]
        n273 = call "IMAQ ArrayToColorImage"("Image Pixels (U32)"=w440, "Image"=w442) -> ("Image Out"=w437:T1)  [unwired: 3 in, 1 out]
        n274 = call "IMAQ ImageToArray"("Image"=w430) -> ("Image Pixels (I16)"=w447:i16[][])  [unwired: 3 in, 4 out]
        n275 = Add(x=w447, y=32768) -> (x+y=w445:i32[][])
        n276 = To Unsigned Word Integer(number=w445) -> (unsigned 16bit integer=w435:u16[][])
        n277 = To Unsigned Long Integer(number=w435) -> ()  [unwired: 1 out]
        n278 = case shown="False" w454 {
          tunnel: w455 -> [w461 w462]
          tunnel: [w460 w462] -> w450
          frame False {
            n279 = Create Folder(path (use dialog)=w461) -> (created path=w460:path)  [unwired: 2 in, 2 out]
          }
          frame True {
          }
        }
        n280 = call "IMAQ ArrayToImage"("Image Pixels (U16)"=w435, "Image"=w425) -> ("Image Out"=w419:T1)  [unwired: 8 in, 1 out]
        n281 = Build Path(base path=w450, name or relative path="ExportImage.png") -> (appended path=w423:path)
        n282 = call "IMAQ Cast Image"("Image Type"=w432, "# Shifts"="# Shifts", "Image Dst"=w426, "Image Src"=w419) -> ("Image Dst Out"=w418:T1)  [unwired: 6 in, 1 out]
        n283 = call "IMAQ Multiply"("Image Src A"=w418, "Constant"="Constant", "Image Dst"=w418) -> ("Image Dst Out"=w416:T1)  [unwired: 4 in, 1 out]
        n284 = call "IMAQ ReplaceColorPlane"("Image Src"=w437, "Color Mode"=w436, "Image Dst"=w437, "Red or Hue Plane"=w416, "Green or Sat Plane"=w416, "Blue or Luma or Val or Inten Plane"=w416) -> ("Image Dst Out"=w428:T1)  [unwired: 8 in, 1 out]
        "Image Out" <- w428
        n285 = call "IMAQ Copy Overlay"("Groups"=w429, "Image Dst"=w428, "Image Src"=w430) -> ("error out"=w427:errorcluster)  [unwired: 7 in, 1 out]
        n286 = call "IMAQ Merge Overlay"("Groups"=w429, "error in (no error)"=w427, "Image Dst"=w428, "Image Src"=w428) -> ("error out"=w422:errorcluster, "Image Dst Out"=w421:T1)  [unwired: 6 in]
        n287 = call "IMAQ Write Image And Vision Info File 2"("error in (no error)"=w422, "File Path"=w423, "Image"=w421) -> ("error out"=w420:errorcluster)  [unwired: 7 in, 1 out]
        n288 = case shown="No Error" w420 {
          tunnel: w426 -> [w459 _]
          tunnel: w425 -> [w458 _]
          tunnel: w424 -> [w457 _]
          frame No Error {
            n289 = call "IMAQ Dispose"("Image"=w457) -> ()  [unwired: 5 in, 1 out]
            n290 = call "IMAQ Dispose"("Image"=w458) -> ()  [unwired: 5 in, 1 out]
            n291 = call "IMAQ Dispose"("Image"=w459) -> ()  [unwired: 5 in, 1 out]
          }
          frame Error {
          }
        }
      }
    }
  }
  n292 = call "IMAQ Dispose"("All Images? (No)"=TRUE, "Image"=w28, "error in (no error)"=w30) -> ()  [unwired: 3 in, 1 out]
  n293 = call "IMAQ Dispose"("Image"=w24) -> ()  [unwired: 5 in, 1 out]
